vi "Polynomial Interpolation PtByPt.vi"(0 "y":dbl format="%0.2f", 1 "x":dbl format="%0.2f", 2 "sample length":i32=10, 3 "x value":dbl format="%0.2f", 4 "initialize":bool) -> (5 "interpolation value":dbl format="%0.2f", 6 "interpolation error":dbl format="%0.2f", 7 "error":i32)   [LabVIEW 2020, in "NI_PtbyPt.lvlib"]
doc: "Interpolates or extrapolates the function f at <B>x</B>."
uses:
  <vilib>/ptbypt/NI_PtbyPt.lvlib
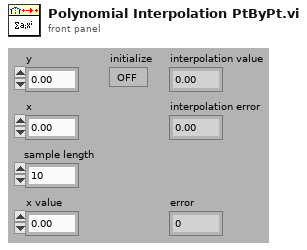
[diagram p1: front panel]
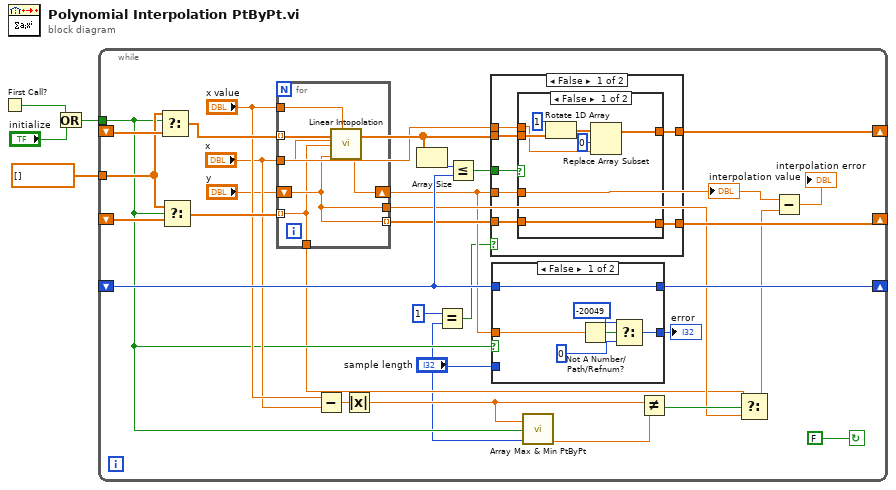
[diagram p0: block diagram]
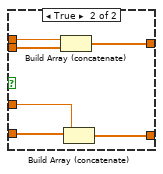
[diagram p2: hidden frame]
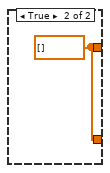
[diagram p3: hidden frame]
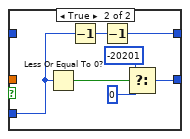
[diagram p4: hidden frame]
diagram:
  n1 = First Call?() -> (First Call?: T/F=w4:bool)
  n2 = Or(x=w4, y="initialize") -> (x .or. y?=w2:bool)
  n3 = while {
    shift-left: _ -> [w26]
    shift-right: [w27] -> _
    tunnel: dbl[] [] ("t") -> [w31]
    tunnel: w2 -> [w12]
    shift-left: _ -> [w33]
    shift-right: [w21] -> _
    shift-left: _ -> [w32]
    shift-right: [w34] -> _
    stop <- FALSE continue-if-true
    n4 = Select(t=w31, s=w12, f=w32) -> (s? t:f=w29:dbl[])
    n5 = Select(t=w31, s=w12, f=w33) -> (s? t:f=w24:dbl[])
    n6 = for {
      shift-right: [w71] -> w8
      shift-left: "y" -> [w70]
      tunnel: w29 -> [w74] mode=indexing
      tunnel: "x" -> [w73]
      tunnel: w24 -> [w69] mode=indexing
      tunnel: "x value" -> [w72]
      tunnel: [w70] -> w22 mode=indexing
      tunnel: [w70] -> w10
      tunnel: [w69] -> w9
      n7 = call <vilib>:"Linear Intopolation.vi"("x1"=w74, "x2"=w73, "y1"=w69, "y2"=w70, "x"=w72) -> ("y"=w71:dbl)
    }
    "interpolation value" <- w8
    n8 = Subtract(x="x value", y="x") -> (x-y=w18:dbl)
    n9 = Absolute Value(x=w18) -> (abs(x)=w14:dbl)
    n10 = Array Size(array=w29) -> (size(s)=w28:i32)
    n11 = Equal?(x=1, y="sample length") -> (x = y?=w5:bool)
    n12 = Less Or Equal?(x=w28, y=w26) -> (x <= y?=w23:bool)
    n13 = case shown="False" w5 {
      tunnel: [w41 w55] -> w34
      tunnel: w29 -> [w40 _]
      tunnel: w23 -> [w39 _]
      tunnel: w22 -> [w38 _]
      tunnel: [w37 w55] -> w21
      tunnel: "x" -> [w36 _]
      tunnel: w8 -> [w35 _]
      frame False {
        n14 = case shown="False" w39 {
          tunnel: [w46 w54] -> w41
          tunnel: w36 -> [w43 w53]
          tunnel: w40 -> [w48 w52]
          tunnel: w38 -> [w42 w51]
          tunnel: w35 -> [_ w50]
          tunnel: [w42 w49] -> w37
          frame False {
            n15 = Rotate 1D Array(1:w48, 2:1 ("n")) -> (0:w45:dbl[])
            n16 = Replace Array Subset(array=w45, new element=w43, index=0 ("Index")) -> (w46:dbl[])
          }
          frame True {
            n17 = Build Array (concatenate)(w53, w52) -> (w54:dbl[])
            n18 = Build Array (concatenate)(w51, w50) -> (w49:dbl[])
          }
        }
      }
      frame True {
        w55 = dbl[] []
      }
    }
    n19 = case shown="False" w12 {
      tunnel: "sample length" -> [_ w64]
      tunnel: [w57 w67] -> w30
      tunnel: w8 -> [w61 _]
      tunnel: [w56 w63] -> w27
      tunnel: w26 -> [w56 _]
      frame False {
        n20 = Not A Number/Path/Refnum?(number/path/refnum=w61) -> (NaN/Path/Refnum?=w60:bool)
        n21 = Select(t=-20049, s=w60, f=0) -> (s? t:f=w57:i32)
      }
      frame True {
        n22 = Less Or Equal To 0?(x=w64) -> (x <= 0?=w68:bool)
        n23 = Decrement(x=w64) -> (x-1=w62:i32)
        n24 = Decrement(x=w62) -> (x-1=w63:i32)
        n25 = Select(t=-20201 ("f"), s=w68, f=0 ("t")) -> (s? t:f=w67:i32)
      }
    }
    "error" <- w30
    n26 = call <vilib>:"Array Max & Min PtByPt.vi"("input data point"=w14, "sample length"="sample length", "initialize"=w12) -> ("min value"=w13:dbl)  [unwired: 4 out]
    n27 = Not Equal?(x=w14, y=w13) -> (x != y?=w16:bool)
    n28 = Select(t=w9, s=w16, f=w10) -> (s? t:f=w17:dbl)
    n29 = Subtract(x=w8, y=w17) -> (x-y=→"interpolation error":dbl)
  }
